vi "Beam Profiler Setup ROI.vi"(0 "Camera Notifier Name":string) -> (8 "Canceled?":bool)   [LabVIEW 2020]
uses:
  <vilib>/Utility/miscctls.llb/LVPointTypeDef.ctl
  Device Library/Cameras/Camera Controls/Generic Camera ROI.ctl
  Device Library/Cameras/Polymorphic Camera Messenger/Set ROI.vi
  Device Library/Cameras/Polymorphic Camera Messenger/Live Preview.vi
  Device Library/Cameras/Polymorphic Camera Messenger/Abort.vi
panel:
  out "ROI Size":string
  in  "Tool Selection":enum32{"Zoom Tool", "ROI Tool", "Pan Tool"}(radio)
  in  "Cancel":bool
  in  "Done":bool
  out "Camera Display":T1(plugin-control)
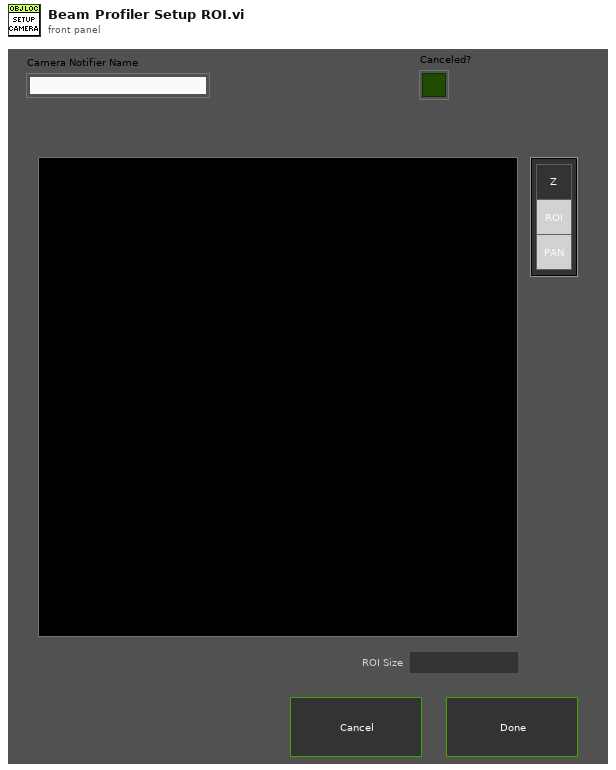
[diagram p1: front panel]
types:
  T1 = typedef "IMAQ Image.ctl" = refnum<image>
  T2 = typedef "Generic Camera ROI.ctl" = cluster{"H_Offset":u16, "V_Offset":u16, "H_Width":u16, "V_Width":u16}
  T3 = enum16{"Always On", "Always Off", "Off While Running"}
  T4 = typedef "LVPointTypeDef.ctl" = cluster{"Horizontal":i16, "Vertical":i16}
  T5 = cluster{"Global Rectangle":i32[], "Contours":cluster{"Contour Type":u32, "ROI Type":u32, "Points":i32[]}[]}
  T6 = cluster{"Contour Type":u32, "ROI Type":u32, "Points":i32[]}[]
  T7 = cluster{"Contour Type":u32, "ROI Type":u32, "Points":i32[]}
  T8 = typedef "LVRectTypeDef.ctl" = cluster{"Left":i16, "Top":i16, "Right":i16, "Bottom":i16}
  T9 = typedef "LVBoundsTypeDef.ctl" = cluster{"Width":u32, "Height":u32}
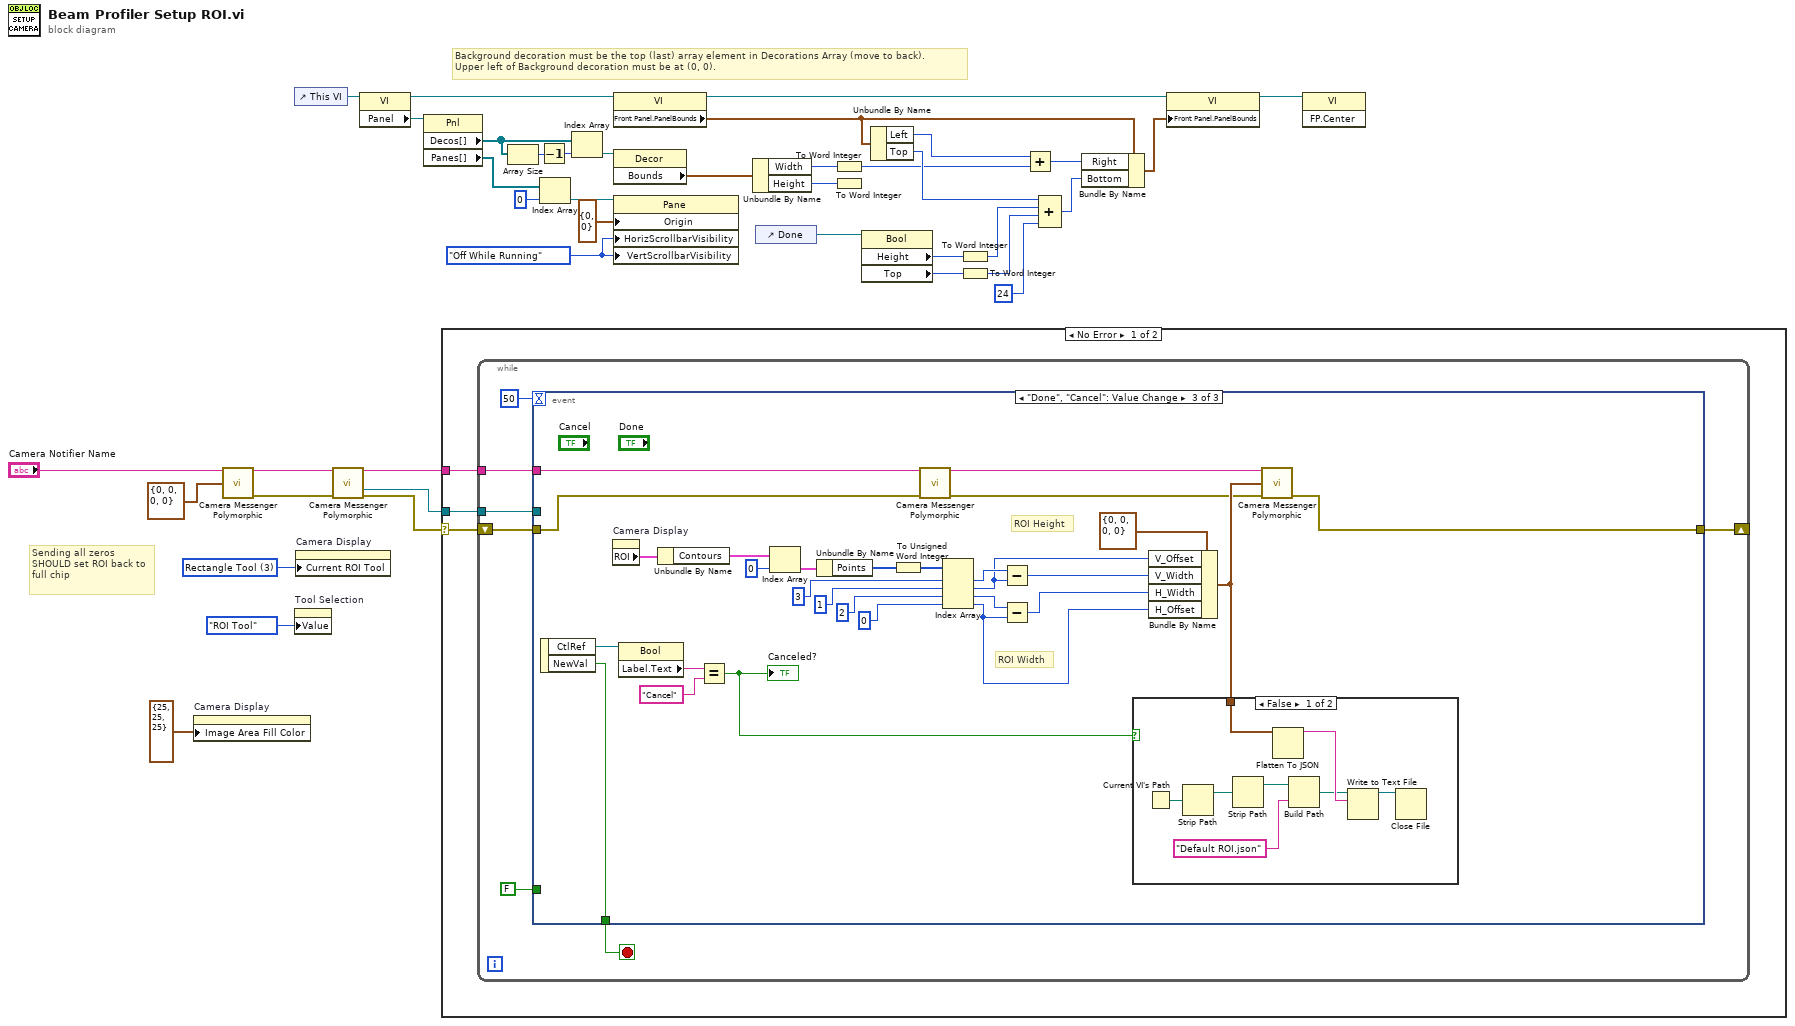
[diagram p0: block diagram]
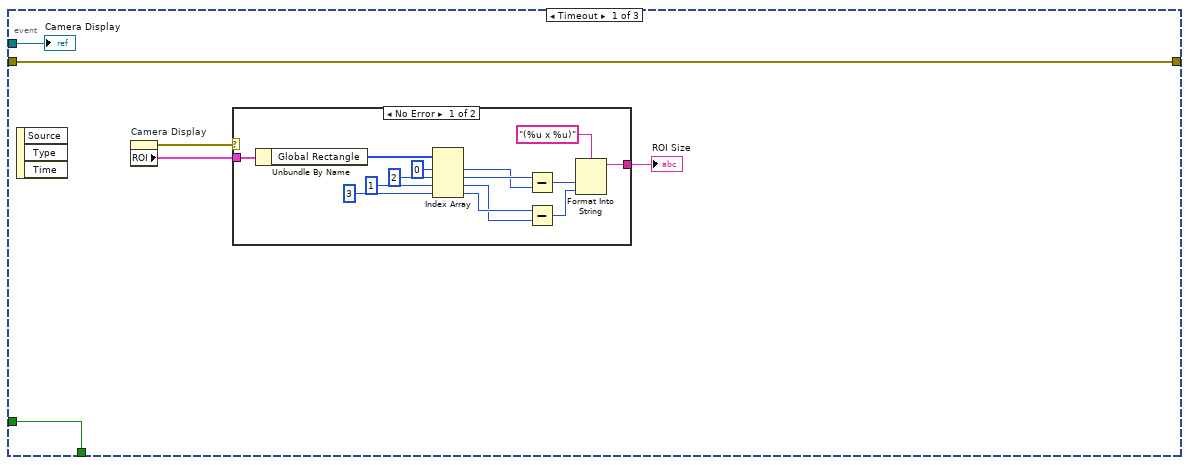
[diagram p2: hidden frame]
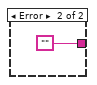
[diagram p3: hidden frame]
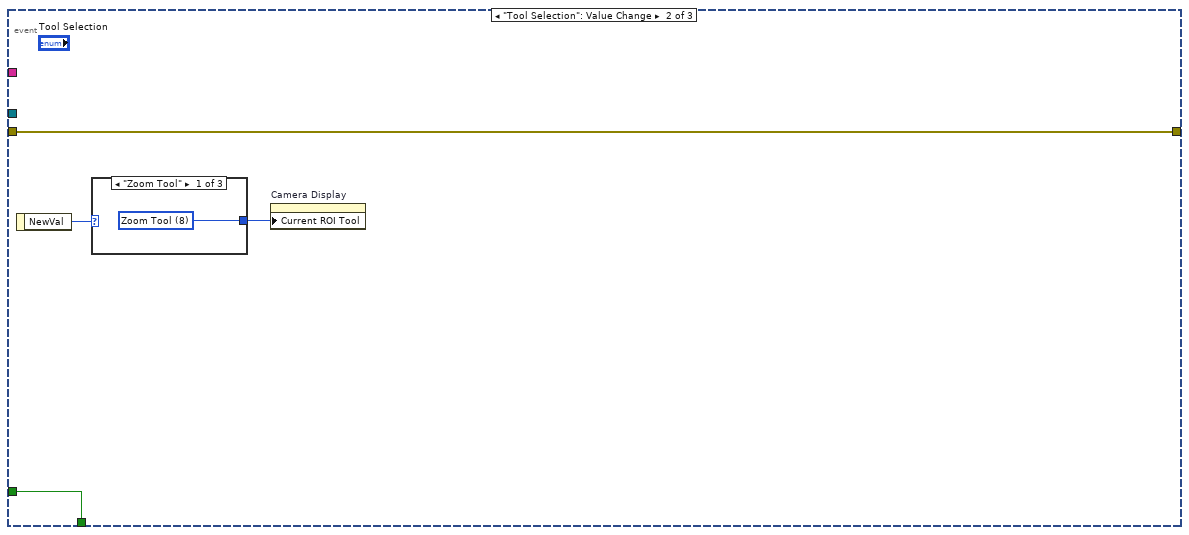
[diagram p4: hidden frame]
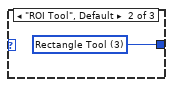
[diagram p5: hidden frame]
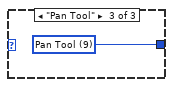
[diagram p6: hidden frame]
diagram:
  w21 = T3."Off While Running" ("Vertical Scrollbar Visibility")
  w40 = u32 3 items=["Zoom Tool"=8, "Selection Tool"=0, "Pan Tool"=9, "Point Tool"=1, "Line Tool"=2, "Rectangle Tool"=3, "Rotated Rectangle Tool"=12, "Polyline Tool"=10, "Polygon Tool"=5, "Freehand Tool"=11, "Closed Freehand Tool"=6, "Ellipse Tool"=4, "Annulus Tool"=7] ("Current ROI Tool")
  # "Background decoration must be the top (last) array element in Decorations Array (move to back).\nUpper left of Background decoration must be at (0, 0)."
  # "Sending all zeros SHOULD set ROI back to full chip"
  n1 = property on="Camera Display" class="ImageControl"("Image Area Fill Color"=cluster{"Red":u8, "Green":u8, "Blue":u8} {"Red"=25, "Green"=25, "Blue"=25} ("Image Area:Background:Background Color")) -> ()  [unwired: 2 in, 2 out]
  n2 = call-poly "Camera Messenger Polymorphic.vi"("Notifier Name"="Camera Notifier Name", "Camera ROI"=T2 {"H_Offset"=0, "V_Offset"=0, "H_Width"=0, "V_Width"=0} ("General Camera ROI")) -> ("Notifier Name DUP"=w6:string, "Error Out"=w3:errorcluster)  [unwired: 12 in]
  n3 = control-ref of="This VI"() -> (w13:refnum<vi>)
  n4 = property on="Tool Selection" class="RadioBtnsControl (strict)"("Value"=enum32{"Zoom Tool", "ROI Tool", "Pan Tool"}."ROI Tool" ("Tool Selection")) -> ()  [unwired: 2 in, 2 out]
  n5 = property on="Camera Display" class="ImageControl"("Current ROI Tool"=w40) -> ()  [unwired: 2 in, 2 out]
  n6 = call-poly "Camera Messenger Polymorphic.vi"("Notifier Name"=w6, "Error In"=w3) -> ("Notifier Name DUP"=w5:string, "Image Ref"=w4:T1, "Error Out"=w2:errorcluster)  [unwired: 10 in, 1 out]
  n7 = property class="VI"(reference=w13) -> (reference out=w22:refnum<vi>, "Panel"=w14:refnum<vi>)  [unwired: 1 in, 1 out]
  n8 = property class="Pnl"(reference=w14) -> ("Decos[]"=w12:refnum<vi>[], "Panes[]"=w18:refnum<vi>[])  [unwired: 1 in, 2 out]
  n9 = case shown="No Error" w2 {
    selector: w2 -> [w41 _]
    tunnel: w5 -> [w43 _]
    tunnel: w4 -> [w42 _]
    frame No Error {
      n10 = while {
        tunnel: w42 -> [w48]
        tunnel: w43 -> [w46]
        shift-right: [w44] -> _
        shift-left: w41 -> [w45]
        stop <- w50 stop-if-true
        n11 = event shown="[2] \"Done\", \"Cancel\": Value Change" {
          selector: _ -> [_ _ _]
          dyn-events: _ -> [_ _ _]
          timeout: 50 -> [_ _ _]
          tunnel: [w56 w75 w103] -> w50
          tunnel: FALSE -> [w56 w75 _]
          tunnel: w48 -> [w55 _ _]
          tunnel: w46 -> [_ _ w84]
          tunnel: w45 -> [w51 w72 w81]
          tunnel: [w51 w72 w79] -> w44
          event Timeout {
            n12 = event-data() -> ()  [unwired: 1 in, 3 out]
            n13 = property on="Camera Display" class="ImageControl"() -> (error out=w53:errorcluster, "ROI"=w54:T5)  [unwired: 2 in, 1 out]
            n14 = case shown="No Error" w53 {
              tunnel: w54 -> [w61 _]
              tunnel: [w57 ""] -> w52
              frame No Error {
                n15 = Unbundle By Name(w61) -> ("Global Rectangle"=w70:i32[])
                n16 = Index Array(array=w70, index #1=0 ("index"), index #2=2 ("index"), index #3=1 ("index"), index #4=3 ("index")) -> (element #1=w64:i32, element #2=w65:i32, element #3=w62:i32, element #4=w63:i32)
                n17 = Subtract(x=w65, y=w64) -> (x-y=w59:i32)
                n18 = Subtract(x=w63, y=w62) -> (x-y=w58:i32)
                n19 = Format Into String(format string="(%u x %u)", w59, w58) -> (resulting string=w57:string)  [unwired: 2 in, 1 out]
              }
              frame Error {
              }
            }
            "ROI Size" <- w52
            "Camera Display" <- w55
          }
          event "Tool Selection": Value Change {
            n20 = event-data() -> ("NewVal"=w74:enum32{"Zoom Tool", "ROI Tool", "Pan Tool"})  [unwired: 1 in]
            n21 = case shown="\"Zoom Tool\"" w74 {
              tunnel: [w76 w77 w78] -> w73
              frame "Zoom Tool" {
                w76 = u32 8 items=["Zoom Tool"=8, "Selection Tool"=0, "Pan Tool"=9, "Point Tool"=1, "Line Tool"=2, "Rectangle Tool"=3, "Rotated Rectangle Tool"=12, "Polyline Tool"=10, "Polygon Tool"=5, "Freehand Tool"=11, "Closed Freehand Tool"=6, "Ellipse Tool"=4, "Annulus Tool"=7] ("Current ROI Tool")
              }
              frame "ROI Tool", Default {
                w77 = u32 3 items=["Zoom Tool"=8, "Selection Tool"=0, "Pan Tool"=9, "Point Tool"=1, "Line Tool"=2, "Rectangle Tool"=3, "Rotated Rectangle Tool"=12, "Polyline Tool"=10, "Polygon Tool"=5, "Freehand Tool"=11, "Closed Freehand Tool"=6, "Ellipse Tool"=4, "Annulus Tool"=7] ("Current ROI Tool")
              }
              frame "Pan Tool" {
                w78 = u32 9 items=["Zoom Tool"=8, "Selection Tool"=0, "Pan Tool"=9, "Point Tool"=1, "Line Tool"=2, "Rectangle Tool"=3, "Rotated Rectangle Tool"=12, "Polyline Tool"=10, "Polygon Tool"=5, "Freehand Tool"=11, "Closed Freehand Tool"=6, "Ellipse Tool"=4, "Annulus Tool"=7] ("Current ROI Tool")
              }
            }
            n22 = property on="Camera Display" class="ImageControl"("Current ROI Tool"=w73) -> ()  [unwired: 2 in, 2 out]
          }
          event "Done", "Cancel": Value Change {
            # "ROI Width"
            # "ROI Height"
            n23 = event-data() -> ("CtlRef"=w106:refnum<vi>, "NewVal"=w103:bool)  [unwired: 1 in]
            n24 = property on="Camera Display" class="ImageControl"() -> ("ROI"=w99:T5)  [unwired: 2 in, 2 out]
            n25 = property class="Bool"(reference=w106) -> ("Label.Text"=w105:string)  [unwired: 1 in, 2 out]
            n26 = Unbundle By Name(w99) -> ("Contours"=w98:T6)
            n27 = Equal?(x=w105, y="Cancel") -> (x = y?=w85:bool)
            "Canceled?" <- w85
            n28 = Index Array(array=w98, index=0) -> (element=w97:T7)
            n29 = Unbundle By Name(w97) -> ("Points"=w100:i32[])
            n30 = To Unsigned Word Integer(number=w100) -> (unsigned 16bit integer=w90:u16[])
            n31 = call-poly "Camera Messenger Polymorphic.vi"("Notifier Name"=w84, "Error In"=w81) -> ("Notifier Name DUP"=w83:string, "Error Out"=w80:errorcluster)  [unwired: 10 in, 2 out]
            n32 = Index Array(array=w90, index #1=3 ("index"), index #2=1 ("index"), index #3=2 ("index"), index #4=0 ("index")) -> (element #1=w102:u16, element #2=w88:u16, element #3=w101:u16, element #4=w89:u16)
            n33 = Subtract(x=w102, y=w88) -> (x-y=w87:u16)
            n34 = Subtract(x=w101, y=w89) -> (x-y=w86:u16)
            n35 = Bundle By Name(cluster=T2 {"H_Offset"=0, "V_Offset"=0, "H_Width"=0, "V_Width"=0} ("General Camera ROI"), "V_Offset"=w88, "V_Width"=w87, "H_Width"=w86, "H_Offset"=w89) -> (w82:T2)
            n36 = case shown="False" w85 {
              tunnel: w82 -> [w110 _]
              frame False {
                n37 = Current VI's Path() -> (path=w109:path)
                n38 = Strip Path(path=w109) -> (stripped path=w108:path)  [unwired: 1 out]
                n39 = Strip Path(path=w108) -> (stripped path=w107:path)  [unwired: 1 out]
                n40 = Flatten To JSON(anything=w110) -> (JSON string=w113:string)  [unwired: 2 in, 1 out]
                n41 = Build Path(base path=w107, name or relative path="Default ROI.json") -> (appended path=w111:path)
                n42 = Write to Text File(file (use dialog)=w111, text=w113) -> (refnum out=w114:refnum<file>)  [unwired: 2 in, 2 out]
                n43 = Close File(refnum=w114) -> ()  [unwired: 1 in, 2 out]
              }
              frame True {
              }
            }
            n44 = call-poly "Camera Messenger Polymorphic.vi"("Notifier Name"=w83, "Camera ROI"=w82, "Error In"=w80) -> ("Error Out"=w79:errorcluster)  [unwired: 11 in, 1 out]
          }
        }
      }
    }
    frame Error {
    }
  }
  n45 = Array Size(array=w12) -> (size(s)=w10:i32)
  n46 = Decrement(x=w10) -> (x-1=w11:i32)
  n47 = Index Array(array=w18, index=0) -> (element=w17:refnum<vi>)
  n48 = Index Array(array=w12, index=w11) -> (element=w20:refnum<vi>)
  n49 = property class="VI"(reference=w22) -> (reference out=w24:refnum<vi>, "Front Panel.PanelBounds"=w25:T8)  [unwired: 1 in, 1 out]
  n50 = property class="Decor"(reference=w20) -> ("Bounds"=w23:T9)  [unwired: 1 in, 2 out]
  n51 = property class="Pane"(reference=w17, "Origin"=T4 {"Horizontal"=0, "Vertical"=0}, "HorizScrollbarVisibility"=w21, "VertScrollbarVisibility"=w21) -> ()  [unwired: 1 in, 2 out]
  n52 = Unbundle By Name(w23) -> ("Width"=w28:u32, "Height"=w31:u32)
  n53 = control-ref of="Done"() -> (w15:refnum<vi>)
  n54 = To Word Integer(number=w28) -> (16bit integer=w30:i16)
  n55 = To Word Integer(number=w31) -> ()  [unwired: 1 out]
  n56 = property class="Bool"(reference=w15) -> ("Height"=w33:u32, "Top"=w34:i32)  [unwired: 1 in, 2 out]
  n57 = Unbundle By Name(w25) -> ("Left"=w27:i16, "Top"=w38:i16)
  n58 = To Word Integer(number=w33) -> (16bit integer=w36:i16)
  n59 = To Word Integer(number=w34) -> (16bit integer=w37:i16)
  n60 = Add(x=w27, y=w30) -> (x+y=w29:i16)
  n61 = Compound Arithmetic op=ADD(w38, w36, w37, i16 24 ("y")) -> (w32:i16)
  n62 = Bundle By Name(cluster=w25, "Right"=w29, "Bottom"=w32) -> (w26:T8)
  n63 = property class="VI"(reference=w24, "Front Panel.PanelBounds"=w26) -> (reference out=w9:refnum<vi>)  [unwired: 1 in, 1 out]
  n64 = invoke class="VI" method="FP.Center"(reference=w9) -> ()  [unwired: 2 in, 3 out]
